vi "Execute Initial Value Policy.vi"(8 "error in (no error)":errorcluster, 9 "Last Publish Time":timestamp, 10 "Last Topic Value":variant, 11 "BasicSubscription In":refnum<class "BasicSubscription.lvclass">) -> (0 "error out":errorcluster, 3 "BasicSubscription Out":refnum<class "BasicSubscription.lvclass">)   [LabVIEW 2018, in "MVA Framework.lvlib" / "SubscriptionPolicy.lvlib" / "BasicSubscription.lvclass"]
doc: "执行初始值策略"
uses:
  BasicSubscription.lvclass
  IMediator/ISubscriptionPolicy/ISubscriptionPolicy.lvclass
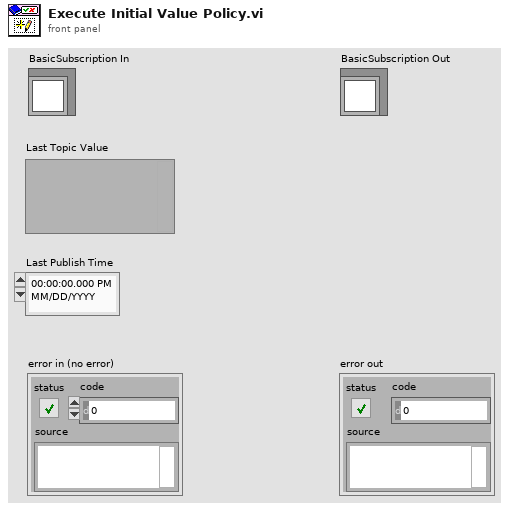
[diagram p1: front panel]
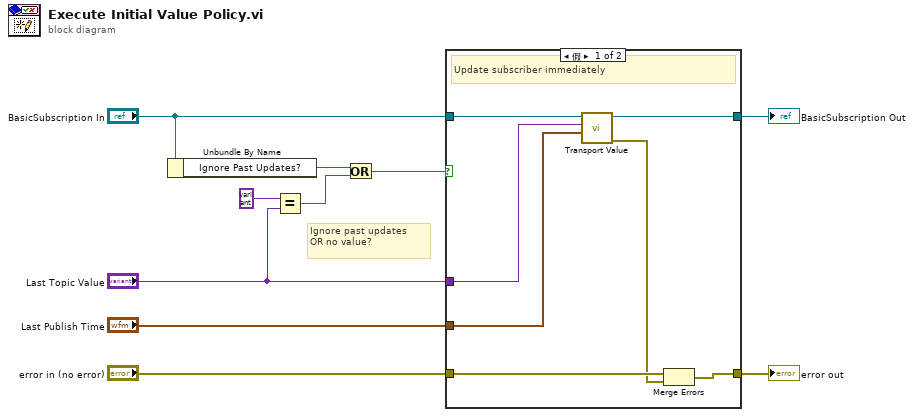
[diagram p0: block diagram]
diagram:
  # "Ignore past updates\nOR no value?"
  n1 = Unbundle By Name("BasicSubscription In") -> ("Ignore Past Updates?"=w3:bool)
  n2 = Equal?(x=variant, y="Last Topic Value") -> (x = y?=w4:bool)
  n3 = Or(x=w3, y=w4) -> (x .or. y?=w2:bool)
  n4 = case shown="假" w2 {
    tunnel: "error in (no error)" -> [w17 w18]
    tunnel: "Last Topic Value" -> [w12 _]
    tunnel: "Last Publish Time" -> [w11 _]
    tunnel: [w16 w18] -> w8
    tunnel: "BasicSubscription In" -> [w15 w19]
    tunnel: [w14 w19] -> w7
    frame False {
      # "Update subscriber immediately"
      n5 = call "Transport Value.vi"("Publish Time"=w11, "Value"=w12, "ISubscriptionPolicy in"=w15) -> ("error out"=w13:errorcluster, "ISubscriptionPolicy out"=w14:refnum<class "BasicSubscription.lvclass">)  [unwired: 7 in]
      n6 = Merge Errors(w17, w13) -> (w16:errorcluster)
    }
    frame True {
      # "Ignore past value OR there is no value"
    }
  }
  "error out" <- w8
  "BasicSubscription Out" <- w7
